vi "Digital_Counter_w_External_Clock.vi"() -> ()   [LabVIEW 2020]
doc: "I. Description:\nThis example demonstrates how to generate a finite digital pulse train from a Counter to be used as the clock for Analog Input.\n\nII. Instructions for Running:\n1. Select the physical channel to correspond to where your signal is input on the DAQ device.\n2. Enter the minimum and maximum signal ranges.\nNote: For better accuracy, try to match the input range to the expected voltage level of the measured signal.\n3. Select the Counter Channel which corresponds to the counter you want to generate your AI clock from.\n4. Select the Source of the Clock for the acquisition as the output of the counter you chose in step 3.\n5. Set the Rate. This will define the Frequency for the Pulse Train Generation which in turn defines the Sample Clock Rate for the voltage channel\n6. Enter the number of Samples per Channel to acquire. \n\nIII. Block Diagram Steps:\n1. Create an analog input voltage channel. Also, create a Counter Output channel to produce a Pulse in terms of Frequency. If the Idle State of the pulse is set to low the first transition of the generated signal is from low to high.\n2. Define the parameters for Clock Source to be the output of the counter. Additionally, define the sample mode to be Finite. Also, use the DAQmx Timing VI (Implicit) to configure the pulse train generation to be continuous.\n3. Call the Start VI to begin the acquisition. Note that data will not be acquired until the counter begins the pulse train. Also, call the Start VI to arm the counter and begin the pulse train generation.\n4. Use the Read VI to retrieve the waveform. Set a timeout so an error is returned if the samples are not returned in the specified time limit. Note: This example reads data from one or more channels and returns an array of data. Use the Index Array function to access an individual channel of data.\n5. Call the Clear Task VI to clear the counter Task.\n6. Call the Clear Task VI to clear the AI Task.\n7. Use the popup dialog box to display an error if any.\n\nIV. I/O Connections Overview:\nMake sure your signal input terminal matches the Physical Channel I/O control. Note that there is no external wiring necessary to connect the counter output to the AI clock input. For further connection information, refer to your hardware reference manual."
uses:
  <vilib>/Utility/error.llb/DialogType.ctl
  <vilib>/DAQmx/read.llb/DAQmx Read (Counter 1D U32 1Chan NSamp).vi
  <vilib>/DAQmx/create/channels.llb/DAQmx Create Channel (CO-Pulse Generation-Frequency).vi
  <vilib>/DAQmx/configure/timing.llb/DAQmx Timing (Implicit).vi
  <vilib>/DAQmx/create/channels.llb/DAQmx Create Channel (CI-Count Edges).vi
  <vilib>/DAQmx/configure/timing.llb/DAQmx Timing (Sample Clock).vi
  <vilib>/DAQmx/miscellaneous.llb/DAQmx Fill In Error Info.vi
panel:
  out "data":u32[](array[numeric])
  in  "stop":bool
  in  "Input":tag
  in  "edge":i32(ring)=10280 items=["Rising"=10280, "Falling"=10171]
  in  "Clock Source":tag="/Dev1/Ctr0InternalOutput" caption="source"
  in  "Rate (Hz)":dbl=1000.0 format="%0.2f"
  in  "Sample Clock Src":tag="Dev1/ctr0" caption="Counter Channel"
  in  "Samples per Channel":i32=1000
  # "Channel Parameters"
  # "Timing Parameters"
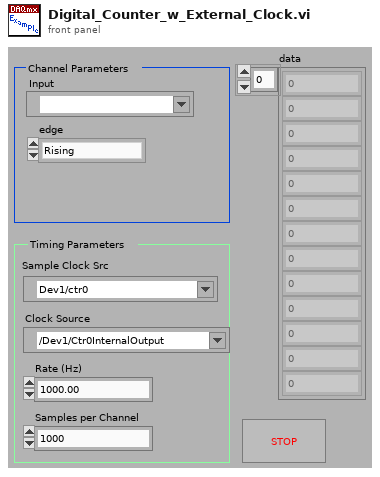
[diagram p1: front panel]
types:
  T1 = typedef "DialogType.ctl" = u16
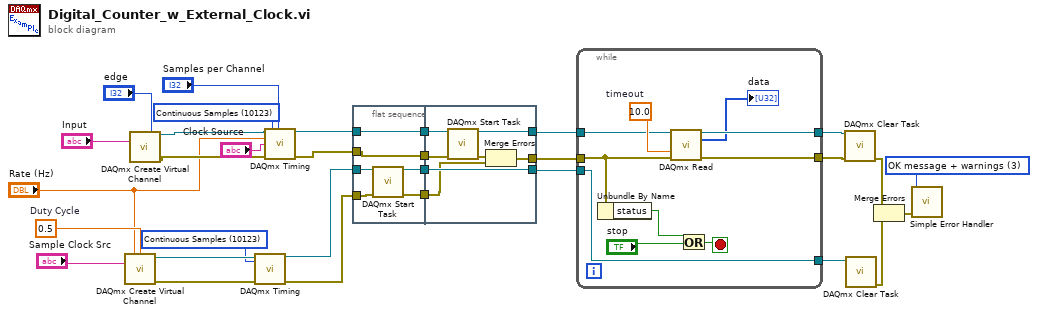
[diagram p0: block diagram]
diagram:
  w24 = T1 3 items=["no dialog", "OK message", "continue or stop message", "OK message + warnings", "continue/stop + warnings"] ("type of dialog (OK msg:1)")
  w27 = 0.5  # Duty Cycle
  w17 = 10123 items=["Finite Samples"=10178, "Continuous Samples"=10123] ("sample mode")
  w29 = 10123 items=["Finite Samples"=10178, "Continuous Samples"=10123] ("sample mode")
  n1 = call-poly <vilib>:"DAQmx Create Virtual Channel.vi"("frequency"="Rate (Hz)", "duty cycle"=w27, "counter"="Sample Clock Src") -> ("task out"=w30:refnum<k21>, "error out"=w31:errorcluster)  [unwired: 11 in]
  n2 = call-poly <vilib>:"DAQmx Create Virtual Channel.vi"("edge"="edge", "counter"="Input") -> ("task out"=w21:refnum<k21>, "error out"=w20:errorcluster)  [unwired: 12 in]
  n3 = call-poly <vilib>:"DAQmx Timing.vi"("task/channels in"=w30, "sample mode"=w29, "error in"=w31) -> ("task out"=w25:refnum<k21>, "error out"=w23:errorcluster)  [unwired: 11 in]
  n4 = call-poly <vilib>:"DAQmx Timing.vi"("task/channels in"=w21, "sample mode"=w17, "samples per channel"="Samples per Channel", "rate"="Rate (Hz)", "source"="Clock Source", "error in"=w20) -> ("task out"=w12:refnum<k21>, "error out"=w10:errorcluster)  [unwired: 8 in]
  n5 = flat-sequence {
    tunnel: w25 -> [w36]
    tunnel: w23 -> [w35]
    tunnel: [w37] -> w15
    tunnel: w12 -> [w34]
    tunnel: [w34] -> w13
    tunnel: [w33] -> w11
    tunnel: w10 -> [w33]
    tunnel: [w32] -> w9
    tunnel: [w44] -> w7
    tunnel: w15 -> [w44]
    tunnel: [w43] -> w14
    tunnel: w13 -> [w42]
    tunnel: w11 -> [w41]
    tunnel: w9 -> [w40]
    tunnel: [w38] -> w2
    frame #0 {
      n6 = call <vilib>:"DAQmx Start Task.vi"("task/channels in"=w36, "error in"=w35) -> ("task out"=w37:refnum<k21>, "error out"=w32:errorcluster)  [unwired: 12 in]
    }
    frame #1 {
      n7 = call <vilib>:"DAQmx Start Task.vi"("task/channels in"=w42, "error in"=w41) -> ("task out"=w43:refnum<k21>, "error out"=w39:errorcluster)  [unwired: 12 in]
      n8 = Merge Errors(w39, w40) -> (w38:errorcluster)
    }
  }
  n9 = while {
    tunnel: w14 -> [w51]
    tunnel: [w54] -> w26
    tunnel: [w50] -> w8
    tunnel: w7 -> [w46]
    tunnel: w2 -> [w45]
    tunnel: [w46] -> w1
    stop <- w49 stop-if-true
    w52 = 10.0  # timeout
    n10 = Unbundle By Name(w45) -> ("status"=w48:bool)
    n11 = call-poly <vilib>:"DAQmx Read.vi"("task/channels in"=w51, "timeout"=w52, "error in"=w45) -> ("task out"=w54:refnum<k21>, "data"=→"data":u32[], "error out"=w50:errorcluster)  [unwired: 10 in]
    n12 = Or(x=w48, y="stop") -> (x .or. y?=w49:bool)
  }
  n13 = call <vilib>:"DAQmx Clear Task.vi"("task in"=w26, "error in"=w8) -> ("error out"=w3:errorcluster)  [unwired: 13 in]
  n14 = call <vilib>:"DAQmx Clear Task.vi"("task in"=w1) -> ("error out"=w4:errorcluster)  [unwired: 14 in]
  n15 = Merge Errors(w3, w4) -> (w5:errorcluster)
  n16 = call <vilib>:"Simple Error Handler.vi"("type of dialog (OK msg:1)"=w24, "error in (no error)"=w5) -> ()  [unwired: 3 in, 5 out]
